vi "Find Available Cells.vi"(0 "Input Parsed":T1, 11 "error in (no error)":errorcluster) -> (4 "Board Available":bool[][](array[boolean]), 15 "error out":errorcluster)   [LabVIEW 2014, in "Dragon Tamers.lvlib"]
uses:
  Dragon Tamers.lvlib
  Typedefs/Input Parsed.ctl
  Typedefs/King.ctl
  Typedefs/Cell Pos.ctl
  Typedefs/Board.ctl
  Typedefs/Board Cell.ctl
  Typedefs/Cell Occupancy.ctl
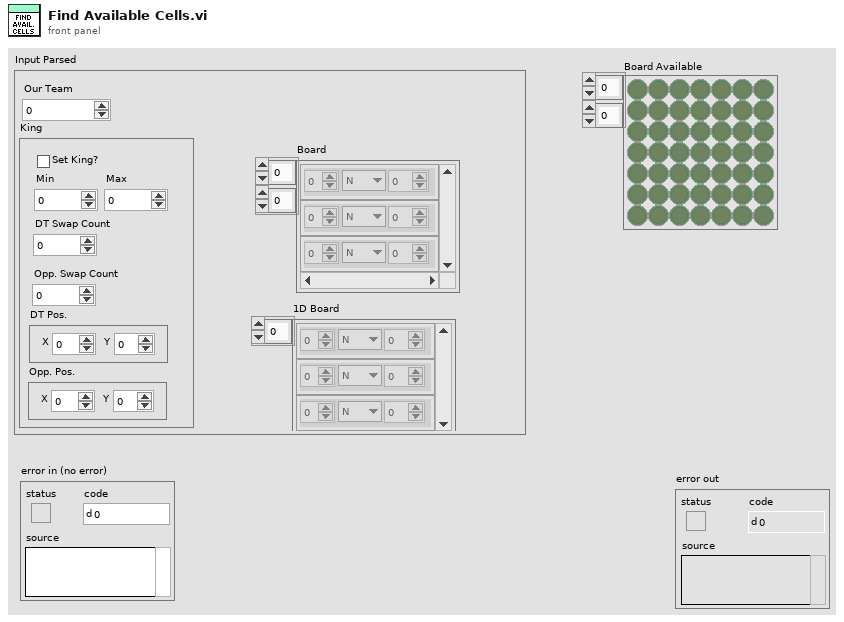
[diagram p1: front panel]
types:
  T1 = typedef "Dragon Tamers.lvlib/Input Parsed.ctl" = cluster{"Our Team":i32, "King":T2, "Board":T4, "1D Board":T5[]}
  T2 = typedef "Dragon Tamers.lvlib/King.ctl" = cluster{"Set King?":bool, "Min":i32, "Max":i32, "DT Swap Count":i32, "Opp. Swap Count":i32, "DT Pos.":T3, "Opp. Pos.":T3}
  T3 = typedef "Dragon Tamers.lvlib/Cell Pos.ctl" = cluster{"X":i32, "Y":i32}
  T4 = typedef "Dragon Tamers.lvlib/Board.ctl" = T5[][]
  T5 = typedef "Dragon Tamers.lvlib/Board Cell.ctl" = cluster{"Team":i32, "Occu.":T6, "Count":i32}
  T6 = typedef "Dragon Tamers.lvlib/Cell Occupancy.ctl" = enum16{"N", "C", "K"}
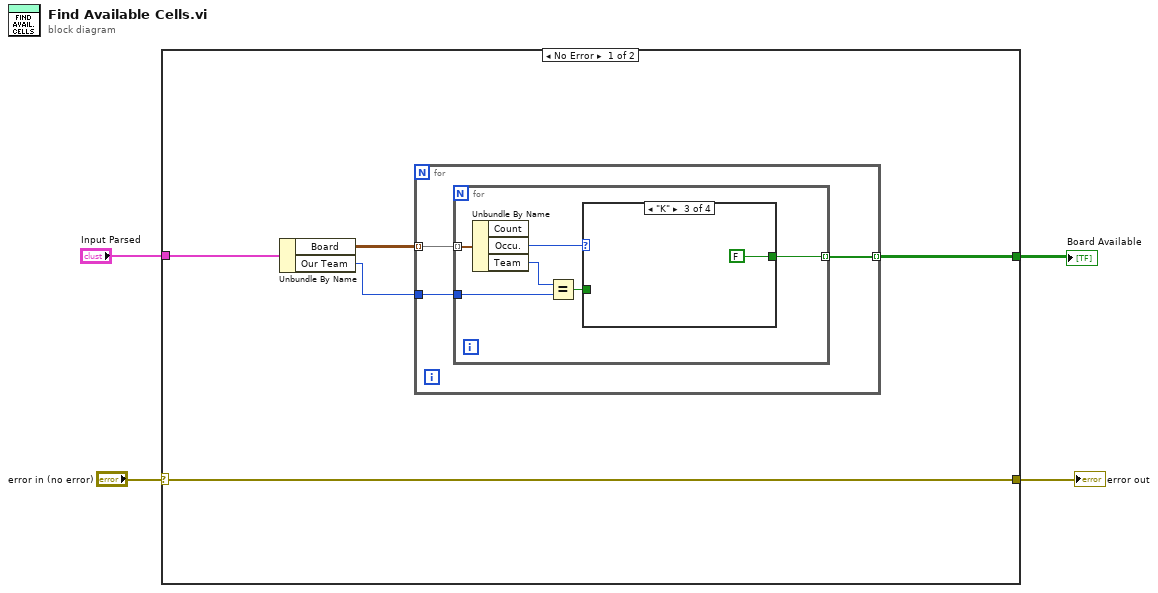
[diagram p0: block diagram]
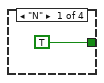
[diagram p2: hidden frame]
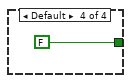
[diagram p4: hidden frame]
diagram:
  n1 = case shown="No Error" "error in (no error)" {
    selector: "error in (no error)" -> [w7 w23]
    tunnel: [w7 w23] -> w3
    tunnel: "Input Parsed" -> [w6 _]
    tunnel: [w5 _] -> w1
    frame No Error {
      n2 = Unbundle By Name(w6) -> ("Board"=w9:T4, "Our Team"=w8:i32)
      n3 = for {
        tunnel: w9 -> [w12] mode=indexing
        tunnel: w8 -> [w11]
        tunnel: [w10] -> w5 mode=indexing
        n4 = for {
          tunnel: w12 -> [w18] mode=indexing
          tunnel: w11 -> [w16]
          tunnel: [w14] -> w10 mode=indexing
          n5 = Unbundle By Name(w18) -> ("Occu."=w15:T6, "Team"=w17:i32)  [unwired: 1 out]
          n6 = Equal?(x=w17, y=w16) -> (x = y?=w13:bool)
          n7 = case shown="\"K\"" w15 {
            tunnel: [TRUE w20 FALSE FALSE] -> w14
            tunnel: w13 -> [_ w20 _ _]
            frame "N" {
            }
            frame "C" {
            }
            frame "K" {
            }
            frame Default {
            }
          }
        }
      }
    }
    frame Error {
    }
  }
  "error out" <- w3
  "Board Available" <- w1
